vi "aceptable.vi"() -> ()   [LabVIEW 2023]
uses:
  <vilib>/Platform/TimedLoop/XDataNode/timing_clust.ctl
  <vilib>/Platform/TimedLoop/XDataNode/nitl_modes.ctl
  <vilib>/Platform/TimedLoop/XDataNode/wakeup.ctl
  <vilib>/addons/control/pid/pid.llb/PID (DBL).vi
  <vilib>/platform/TimedLoop/XDataNode/XDataNode.xnode
  <vilib>/Platform/TimedLoop/XDataNode/XDNodeRunTimeDep.lvlib
  <vilib>/addons/control/pid/NI_PID_pid.lvlib
panel:
  in  "PID gains":T1={"proportional gain (Kc)"=0.0166666666666, "integral time (Ti, min)"=0.01, "derivative time (Td, min)"=0.0}
  out "compraracion sensor-consigna":cluster{"Luz":i32, "ref":dbl}(graph)
  out "Señal PWM":dbl(graph)
  in  "consigna":dbl
  out "error sensor consigna":dbl(graph)
  out "Trama PWM":string
  out "trama completa":string
  out "ind trama":i32
  out "Trama":i32
  out "Resto trama":string
  in  "Puerto":refnum<visa-resource-name>
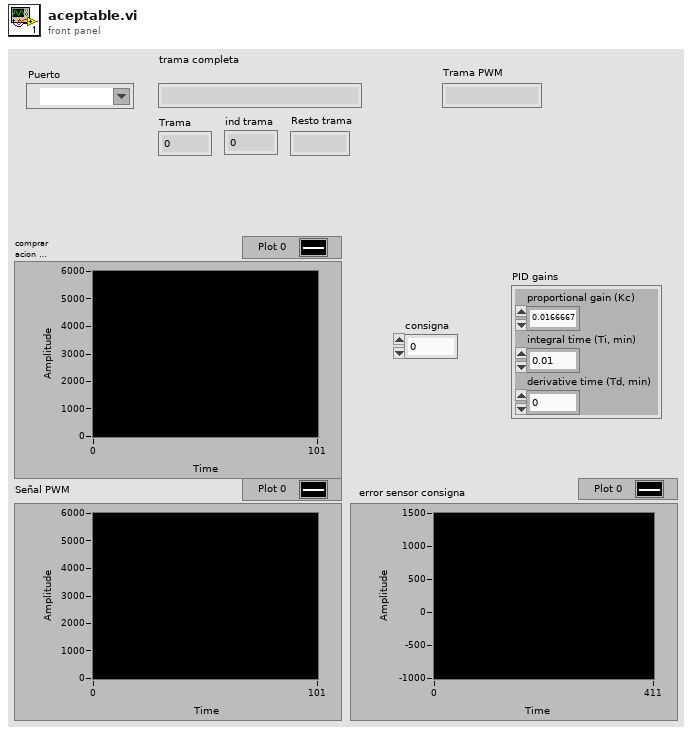
[diagram p1: front panel]
types:
  T1 = cluster{"proportional gain (Kc)":dbl, "integral time (Ti, min)":dbl, "derivative time (Td, min)":dbl}
  T2 = typedef "XDNodeRunTimeDep.lvlib/timing_clust.ctl" = cluster{"Expected End [f-1]":u64, "Actual End [f-1]":u64, "Finished Late? [f-1]":bool, "Expected End [i-1]":u64, "Actual End [i-1]":u64, "Finished Late? [i-1]":bool, "Expected Start [i]":u64, "Actual Start [i]":u64, "Expected Start [f]":u64, "Actual Start [f]":u64, "Source Name":string, "Structure Name":string, "Period":i64, "Deadline":i64, "Offset":i64, "Start":i64, "Priority":i32, "Timeout":i32, "Mode":T3, "Wakeup Reason":T4, "Error":errorcluster, "Source Type":string, "Secondary Source Type":string, "Global End Time":u64, "Global Start Time":u64, "Frame Duration":u64, "Iteration Duration":u64, "Assigned CPU":i32, "I/O Scan Engine Mode":u32}
  T3 = typedef "XDNodeRunTimeDep.lvlib/nitl_modes.ctl" = enum32{"No Change", "Process missed periods, maintain original phase", "Discard missed periods, maintain original phase", "Process missed periods, ignore original phase", "Discard missed periods, ignore original phase"}
  T4 = typedef "XDNodeRunTimeDep.lvlib/wakeup.ctl" = enum32{"Normal", "Aborted", "Asynchronous wakeup", "Timing source error", "Timed loop error", "Timeout"}
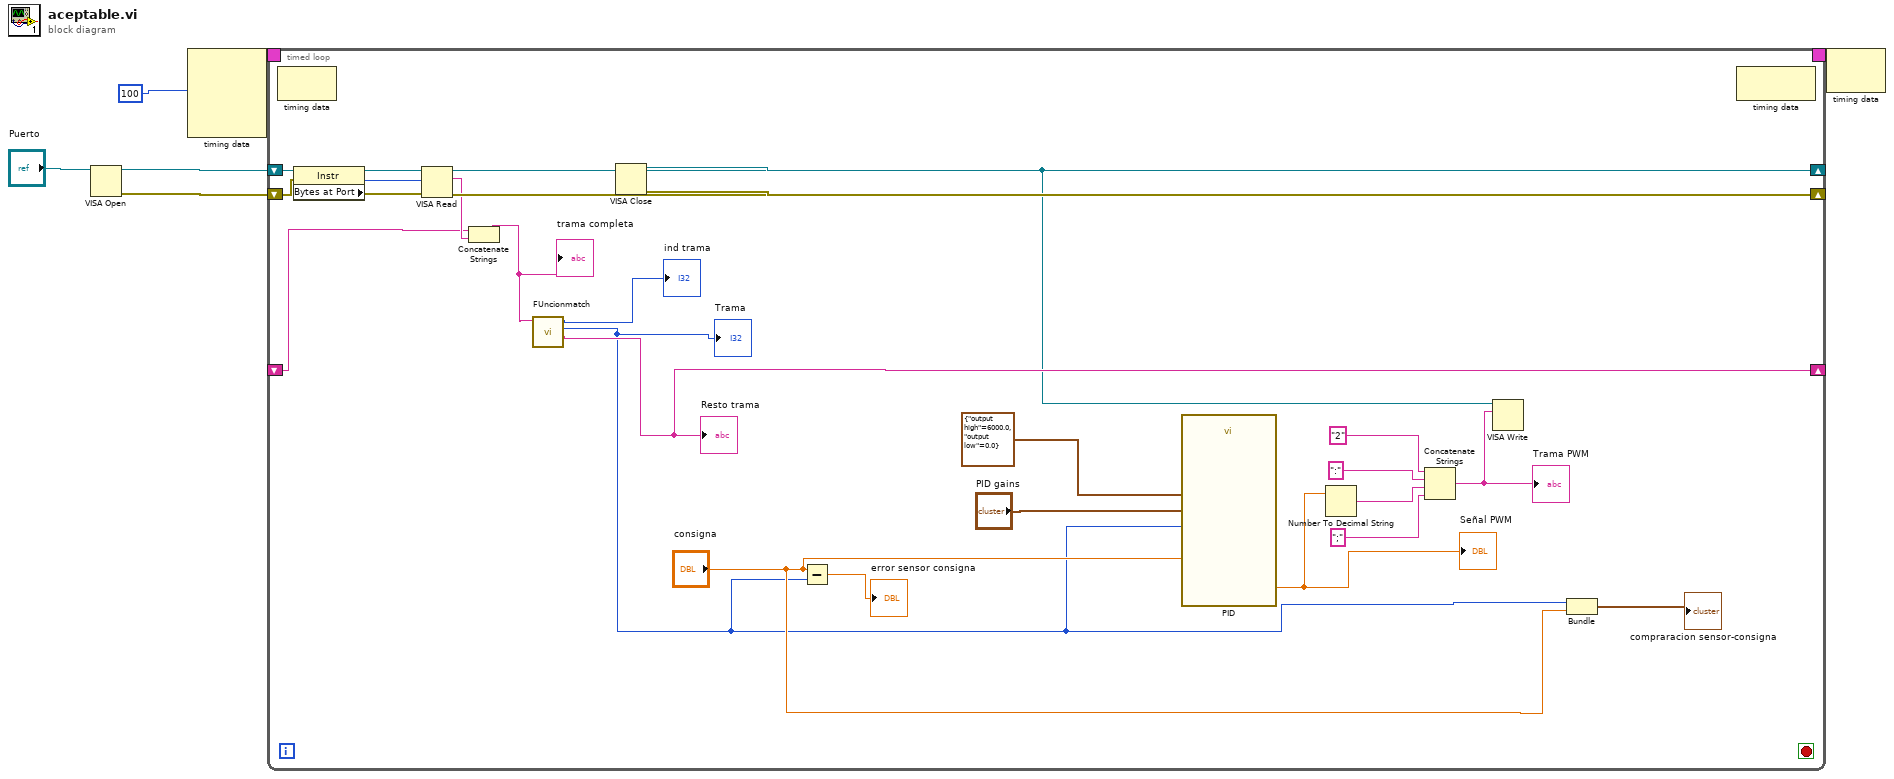
[diagram p0: block diagram]
diagram:
  n1 = VISA Open(VISA resource name="Puerto") -> (VISA resource name=w5:refnum<visa-resource-name>, error out=w4:errorcluster)  [unwired: 4 in]
  n2 = node-c288(i64 100 ("Period")) -> (w8:T2)  [unwired: 3 in]
  n3 = timed-loop {
    timing: w8 -> [_]
    timing-out: [_] -> w7
    shift-right: [w17] -> w2
    shift-left: w5 -> [w32]
    shift-right: [w27] -> w1
    shift-left: w4 -> [w31]
    shift-right: [w23] -> _
    shift-left: _ -> [w22]
    stop <- _ stop-if-true
    n4 = node-c288() -> ()  [unwired: 1 in, 1 out]
    n5 = property class="Instr"(reference=w32, error in=w31) -> (reference out=w30:refnum<visa-resource-name>, error out=w29:errorcluster, "Bytes at Port"=w28:u32)
    n6 = VISA Read(VISA resource name=w30, byte count=w28, error in (no error)=w29) -> (VISA resource name out=w17:refnum<visa-resource-name>, read buffer=w26:string, error out=w27:errorcluster)  [unwired: 1 out]
    n7 = Concatenate Strings(w22, w26) -> (w25:string)
    "trama completa" <- w25
    n8 = call "FUncionmatch.vi"("Entrada"=w25) -> ("Salida"=w23:string, "number 2"=w10:i32, "number"=→"ind trama":i32)  [unwired: 8 in]
    "Trama" <- w10
    "Resto trama" <- w23
    n9 = Subtract(x="consigna", y=w10) -> (x-y=→"error sensor consigna":dbl)
    n10 = call-poly <vilib>:"PID.vi"("output range"=cluster{"output high":dbl, "output low":dbl} {"output high"=6000.0, "output low"=0.0}, "PID gains"="PID gains", "process variable"=w10, "setpoint"="consigna") -> ("output"=w14:dbl)  [unwired: 6 in, 1 out]
    "Señal PWM" <- w14
    n11 = Number To Decimal String(number=w14) -> (decimal integer string=w18:string)  [unwired: 1 in]
    n12 = Concatenate Strings("2", ":", w18, ";") -> (w16:string)
    "Trama PWM" <- w16
    n13 = VISA Write(VISA resource name=w17, write buffer=w16) -> ()  [unwired: 1 in, 3 out]
    n14 = Bundle("number 2"=w10, "consigna"="consigna") -> (→"compraracion sensor-consigna":cluster{"number 2":i32, "consigna":dbl})  [unwired: 1 in]
    n15 = node-c288() -> ()  [unwired: 1 in, 1 out]
  }
  n16 = VISA Close(VISA resource name=w2, error in (no error)=w1) -> ()  [unwired: 1 out]
  n17 = node-c288(w7) -> ()  [unwired: 1 out]
